vi "OP500ZP_BOITE_DIALOGUE.vi"(0 "Enable":bool=TRUE caption="Activer", 5 "error in (no error)":errorcluster caption="entrée d'erreur (pas d'erreur)") -> (11 "Factory Temperature":dbl format="%#g", 12 "Min Cell Temperature":dbl format="%#g", 13 "Max Cell Temperature":dbl format="%#g", 14 "Min Cell Voltage":dbl format="%#g", 15 "Max Cell Voltage":dbl format="%#g", 16 "Battery Voltage":dbl format="%#g", 17 "PARK Mode OK?":bool, 18 "OK":bool, 19 "error out":errorcluster caption="sortie d'erreur")   [LabVIEW 2020]
doc: "Affiche une boîte de dialogue standard qui invite l'utilisateur à entrer des informations, telles qu'un nom d'utilisateur et un mot de passe.\n--------------------\n\nCe VI Express est configuré comme suit :\n\nMessage à afficher à l'utilisateur :Saisir les valeur suivantes :\nLes entrées sont : \nCase à cocher : PARK Mode OK?\nNombre : Battery Voltage\nNombre : Max Cell Voltage\nNombre : Min Cell Voltage\nNombre : Max Cell Temperature\nNombre : Min Cell Temperature\nNombre : Factory Temperature"
panel:
  in  "Factory Temperature":dbl format="%#g"
  in  "Min Cell Temperature":dbl format="%#g"
  in  "Max Cell Temperature":dbl format="%#g"
  in  "Min Cell Voltage":dbl format="%#g"
  in  "Max Cell Voltage":dbl format="%#g"
  in  "Battery Voltage":dbl format="%#g"
  in  "PARK Mode OK?":bool
  out "String":string="Saisir les valeur suivantes :" caption="Chaîne"
  in  "Cancel":bool caption="Annuler"
  in  "OK2":bool
  in  "OK1":bool
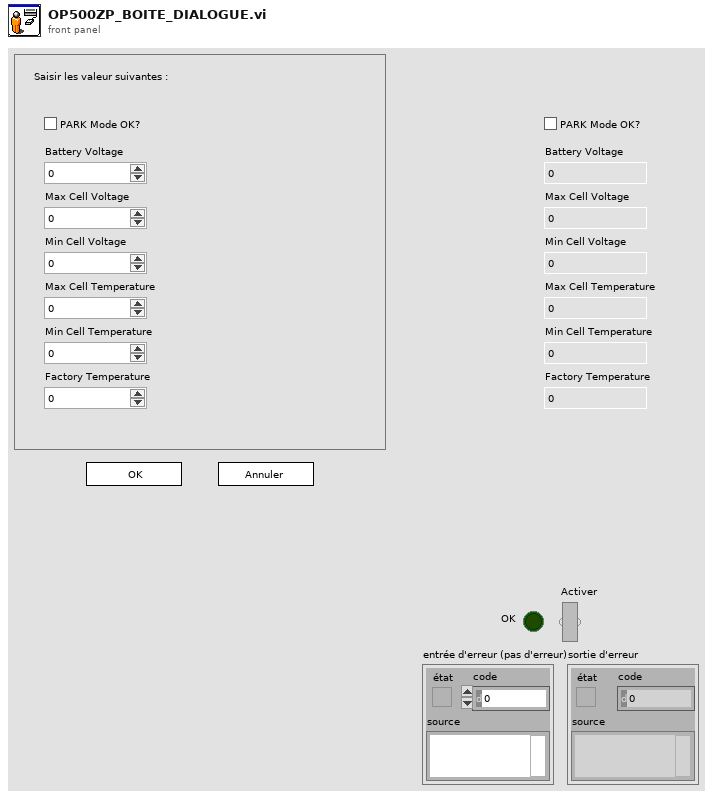
[diagram p1: front panel]
types:
  T1 = cluster{"Input Name":string, "Input Data Type":i32}[]
  T2 = enum8{"Enabled", "Disabled", "Disabled and Grayed Out"}
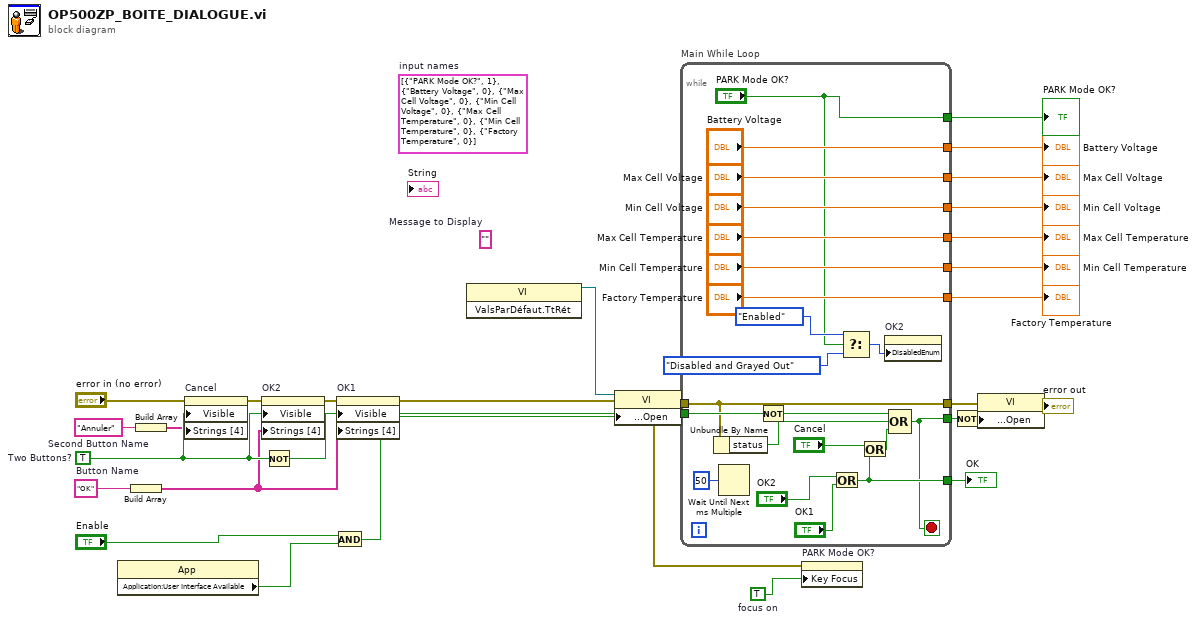
[diagram p0: block diagram]
diagram:
  w9 = TRUE  # focus on
  (unwired) T1 [{"Input Name"="PARK Mode OK?", "Input Data Type"=1}, {"Input Name"="Battery Voltage", "Input Data Type"=0}, {"Input Name"="Max Cell Voltage", "Input Data Type"=0}, {"Input Name"="Min Cell Voltage", "Input Data Type"=0}, {"Input Name"="Max Cell Temperature", "Input Data Type"=0}, {"Input Name"="Min Cell Temperature", "Input Data Type"=0}, {"Input Name"="Factory Temperature", "Input Data Type"=0}]  # input names
  w20 = "Annuler"  # Second Button Name
  w18 = "OK"  # Button Name
  (unwired) ""  # Message to Display
  w28 = TRUE  # Two Buttons?
  n1 = property class="App"() -> ("Application:User Interface Available"=w11:bool)  [unwired: 2 in, 2 out]
  n2 = Build Array(w18) -> (w19:string[])
  n3 = Build Array(w20) -> (w21:string[])
  n4 = property on="Cancel" class="Bool"(error in="error in (no error)", "Visible"=w28, "Strings [4]"=w21) -> (error out=w25:errorcluster)  [unwired: 1 in, 1 out]
  n5 = property on="OK2" class="Bool"(error in=w25, "Visible"=w28, "Strings [4]"=w19) -> (error out=w24:errorcluster)  [unwired: 1 in, 1 out]
  n6 = Not(x=w28) -> (.not. x?=w26:bool)
  n7 = And(x="Enable", y=w11) -> (x .and. y?=w12:bool)
  n8 = property on="OK1" class="Bool"(error in=w24, "Visible"=w26, "Strings [4]"=w19) -> (error out=w1:errorcluster)  [unwired: 1 in, 1 out]
  n9 = invoke class="VI" method="ValsParDéfaut.TtRét"() -> (reference out=w10:refnum<vi>)  [unwired: 3 in, 2 out]
  n10 = property class="VI"(reference=w10, error in=w1, "Front Panel Window:Open"=w12) -> (error out=w17:errorcluster)  [unwired: 1 out]
  n11 = while "Main While Loop" {
    tunnel: [w47] -> w27
    tunnel: w12 -> [w45]
    tunnel: [w43] -> w22
    tunnel: w17 -> [w42]
    tunnel: [w42] -> w15
    tunnel: ["PARK Mode OK?"] -> w2
    tunnel: ["Battery Voltage"] -> w8
    tunnel: ["Max Cell Voltage"] -> w7
    tunnel: ["Min Cell Voltage"] -> w6
    tunnel: ["Max Cell Temperature"] -> w5
    tunnel: ["Min Cell Temperature"] -> w4
    tunnel: ["Factory Temperature"] -> w3
    stop <- w43 stop-if-true
    n12 = Unbundle By Name(w42) -> ("status"=w40:bool)
    n13 = Wait Until Next ms Multiple(millisecond multiple=u32 50) -> ()  [unwired: 1 out]
    n14 = Not(x=w45) -> (.not. x?=w44:bool)
    n15 = Or(x="OK2", y="OK1") -> (x .or. y?=w47:bool)
    n16 = Select(t=T2."Enabled" ("Désactivé"), s="PARK Mode OK?", f=T2."Disabled and Grayed Out" ("Désactivé")) -> (s? t:f=w29:T2)
    n17 = Or(x="Cancel", y=w47) -> (x .or. y?=w41:bool)
    n18 = property on="OK2" class="Bool"("DisabledEnum"=w29) -> ()  [unwired: 2 in, 2 out]
    n19 = Compound Arithmetic op=OR(w44, w40, w41) -> (w43:bool)
  }
  "OK" <- w27
  "PARK Mode OK?" <- w2
  "Battery Voltage" <- w8
  "Max Cell Voltage" <- w7
  "Min Cell Voltage" <- w6
  "Max Cell Temperature" <- w5
  "Min Cell Temperature" <- w4
  "Factory Temperature" <- w3
  n20 = property on="PARK Mode OK?" class="Bool (strict)"(error in=w17, "Key Focus"=w9) -> ()  [unwired: 1 in, 2 out]
  n21 = Not(x=w22) -> (.not. x?=w23:bool)
  n22 = property class="VI"(error in=w15, "Front Panel Window:Open"=w23) -> (error out=→"error out":errorcluster)  [unwired: 1 in, 1 out]
